vi "Find First File Matching Pattern.vi"(8 "error in (no error)":errorcluster, 10 "Patterns":string[](array[string]), 11 "Path":path) -> (0 "error out":errorcluster, 2 "Filename":string)   [LabVIEW 2019, in "Caraya Library.lvlib" / "Caraya Item.lvclass"]
uses:
  Caraya Item.lvclass
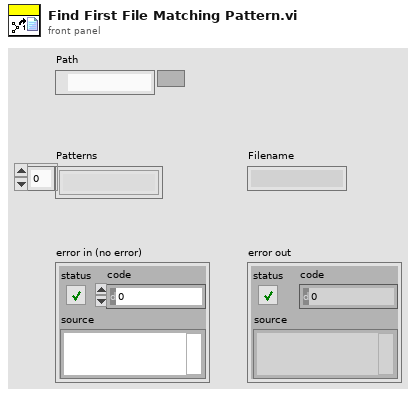
[diagram p1: front panel]
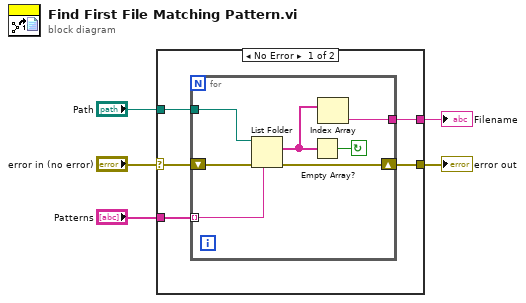
[diagram p0: block diagram]
diagram:
  n1 = case shown="No Error" "error in (no error)" {
    selector: "error in (no error)" -> [w8 w18]
    tunnel: "Patterns" -> [w10 _]
    tunnel: "Path" -> [w9 _]
    tunnel: [w7 w18] -> w2
    tunnel: [w6 _] -> w1
    frame No Error {
      n2 = for {
        tunnel: w10 -> [w17] mode=indexing
        tunnel: w9 -> [w16]
        shift-right: [w14] -> w7
        shift-left: w8 -> [w15]
        tunnel: [w11] -> w6
        stop <- w13 continue-if-true
        n3 = List Folder(path=w16, pattern=w17, error in=w15) -> (filenames=w12:string[], error out=w14:errorcluster)  [unwired: 1 in, 2 out]
        n4 = Empty Array?(array=w12) -> (empty?=w13:bool)
        n5 = Index Array(array=w12) -> (element=w11:string)  [unwired: 1 in]
      }
    }
    frame Error {
    }
  }
  "Filename" <- w1
  "error out" <- w2
